vi "Main.vi"(11 "Module Admin":refnum<class "Delacor_lib_QMH_Module Admin.lvclass">) -> ()   [LabVIEW 2024, in "UI.lvlib"]
doc: "This template is based off of the Queued Message Handler design pattern and the Queued Message Handler project template that ships with LabVIEW.\n\nThe main difference is that the queue is private to this module and communication between modules is performed via Broadcast and Request events.\n\nRequest events are wrapped in public API methods and are handled in the Event Handling Loop (EHL) of this VI. Any module can register for Broadcast events sent by this module. The EHL generates messages based on user interface actions.\n\nThe Message Handling Loop (MHL) processes messages generated by the EHL, or by other messages. The messages are string values, so new messages can be added easily to the Message Cases case structure in the MHL. Each message cluster can also provide an optional value for Message Data, which is a variant that can be converted to whatever message-specific data is required.\n_____\nBased on DQMH Dev Tools: Project Template 7.1.0.1503."
uses:
  UI.lvlib
  <vilib>/Delacor/Delacor QMH/Libraries/Module Admin_class/Delacor_lib_QMH_Module Admin.lvclass
  Module Data--cluster.ctl
  Stop Argument--cluster.ctl
  <vilib>/Delacor/Delacor QMH/Libraries/Message Queue_class/Delacor_lib_QMH_Message Queue.lvclass/Delacor_lib_QMH_Message Queue.ctl
  <vilib>/Delacor/Delacor QMH/Libraries/Module Admin_class/Delacor_lib_QMH_Module Admin.lvclass/Delacor_lib_QMH_Module Admin.ctl
  <vilib>/Delacor/Delacor QMH/Libraries/Message Queue_class/Delacor_lib_QMH_Enqueue Message (Single).vi
  <vilib>/Delacor/Delacor QMH/Libraries/Module Admin_class/Delacor_lib_QMH_Get External Launch.vi
  <vilib>/Delacor/Delacor QMH/Libraries/Message Queue_class/Delacor_lib_QMH_Message Queue.lvclass
  <vilib>/PantherLAB/Message Module/Libraries/Message/PantherLAB_lib_Message.lvlib
  MoneyControl/MoneyControl.lvlib
  ProductControl/ProductControl.lvlib
panel:
  in  "Inventario Listbox":i32(listbox)
  out "Status":string
  in  "Comprar":bool
  out "error out":errorcluster
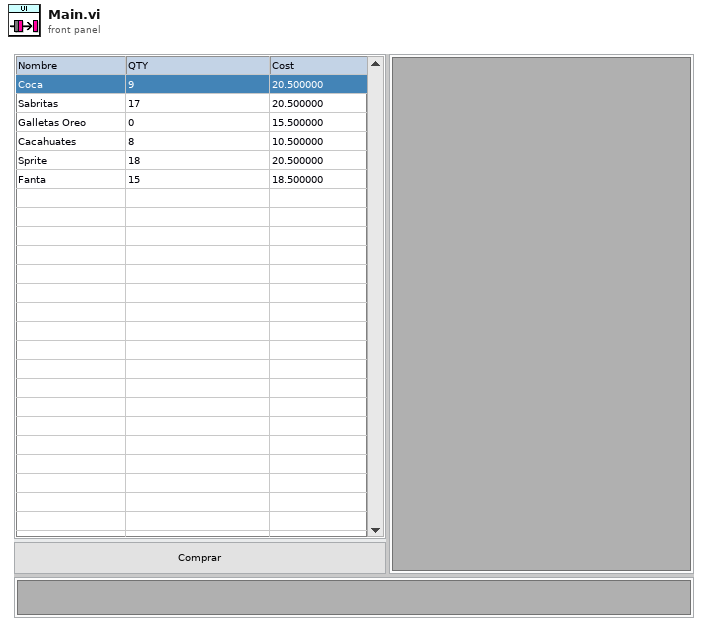
[diagram p1: front panel]
types:
  T1 = typedef "UI.lvlib/Request Events--cluster.ctl" = cluster{"Stop Module":refnum<user-event>, "Show Panel":refnum<user-event>, "Hide Panel":refnum<user-event>, "Get Module Execution Status":refnum<user-event>, "Show Diagram":refnum<user-event>, "Private.Lanza otros modulos":refnum<user-event>}
  T2 = typedef "PantherLAB_lib_Message.lvlib/Broadcast Events--cluster.ctl" = cluster{"Module Did Init":refnum<user-event>, "Status Updated":refnum<user-event>, "Error Reported":refnum<user-event>, "Module Did Stop":refnum<user-event>, "Update Module Execution Status":refnum<user-event>}
  T3 = typedef "MoneyControl.lvlib/Broadcast Events--cluster.ctl" = cluster{"Module Did Init":refnum<user-event>, "Status Updated":refnum<user-event>, "Error Reported":refnum<user-event>, "Module Did Stop":refnum<user-event>, "Update Module Execution Status":refnum<user-event>, "Credito Actualizado":refnum<user-event>, "Cambio Actualizado":refnum<user-event>}
  T4 = typedef "ProductControl.lvlib/Broadcast Events--cluster.ctl" = cluster{"Module Did Init":refnum<user-event>, "Status Updated":refnum<user-event>, "Error Reported":refnum<user-event>, "Module Did Stop":refnum<user-event>, "Update Module Execution Status":refnum<user-event>, "Inventario Actualizado":refnum<user-event>}
  T5 = typedef "UI.lvlib/Module Data--cluster.ctl" = cluster{"Status":string, "Message Module ID":i32}
  T6 = enum32{"invalid lock state", "Not Locked", "Locked (No Password)", "Password-protected"}
  T7 = typedef "UI.lvlib/Stop Argument--cluster.ctl" = cluster{"Origin":string, "Exit via Stop Module Req?":bool, "Wait for Module to stop?":bool}
  T8 = enum32{"Invalid", "Standard", "Closed", "Hidden", "Minimized", "Maximized"}
  T9 = typedef "ProductControl.lvlib/Products--array.ctl" = cluster{"Nombre":string, "QTY":u32, "Value":dbl}[]
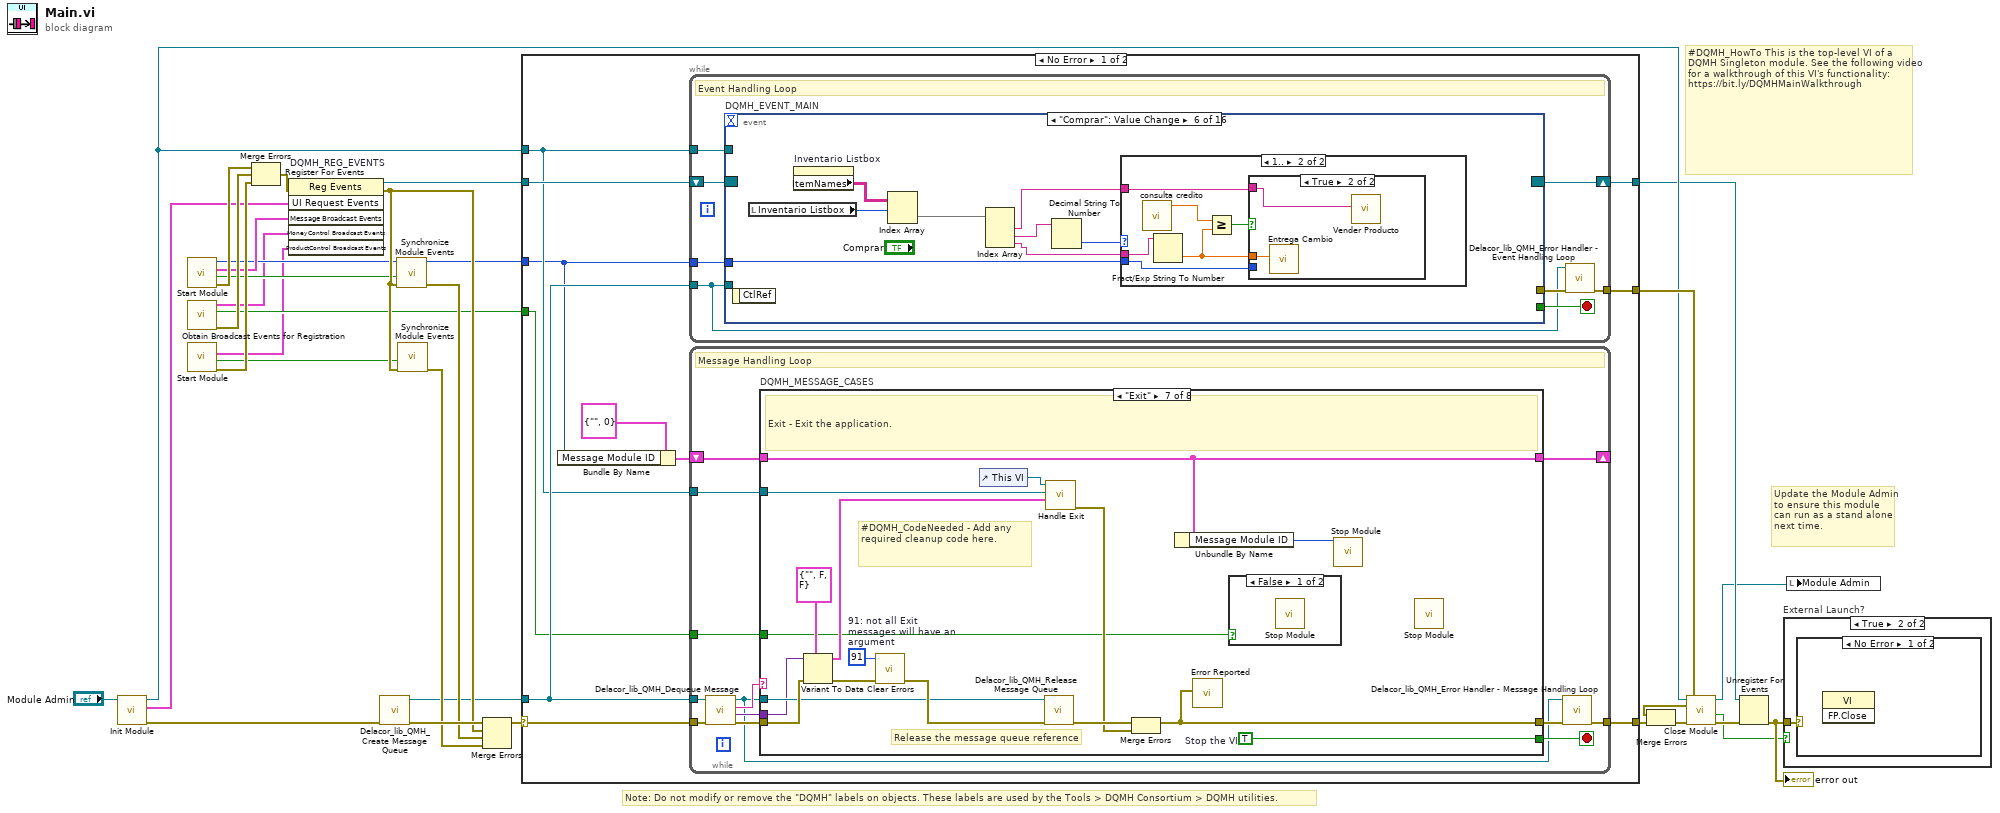
[diagram p0: block diagram]
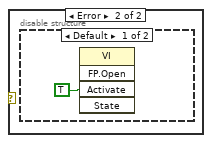
[diagram p3: hidden frame]
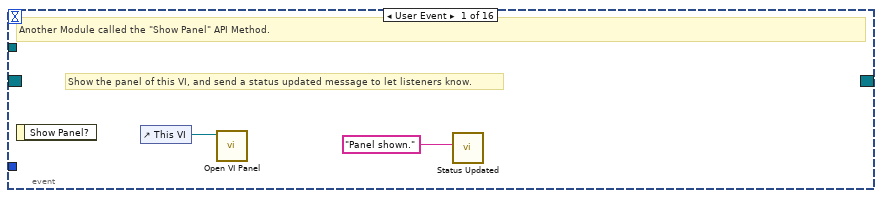
[diagram p5: hidden frame]
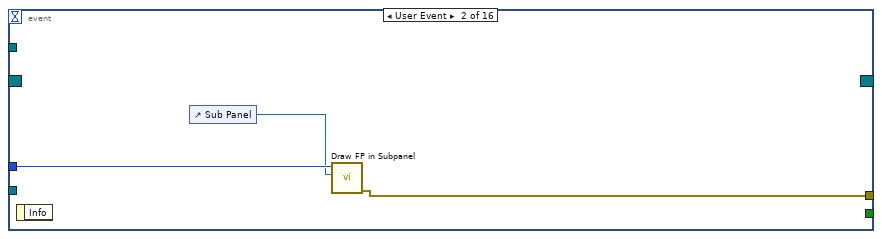
[diagram p6: hidden frame]
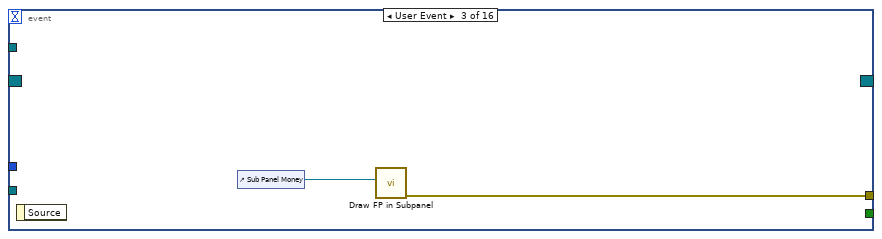
[diagram p7: hidden frame]
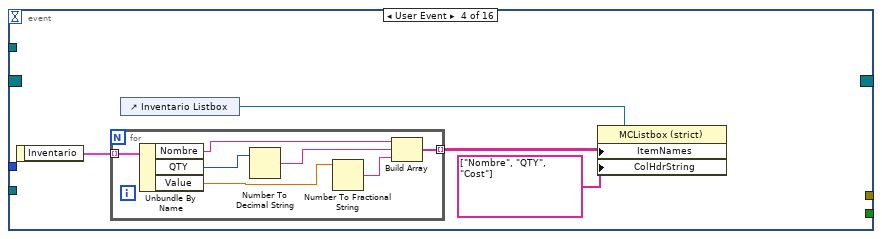
[diagram p8: hidden frame]
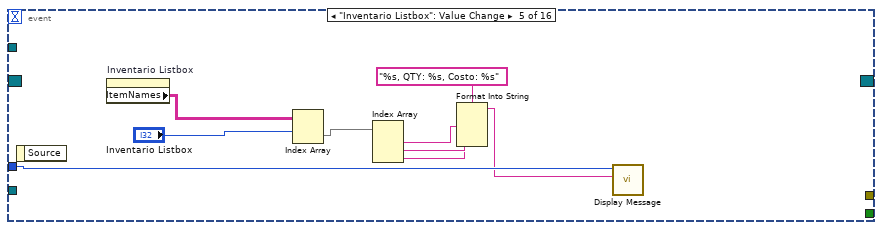
[diagram p9: hidden frame]
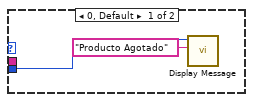
[diagram p10: hidden frame]
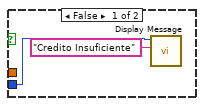
[diagram p11: hidden frame]
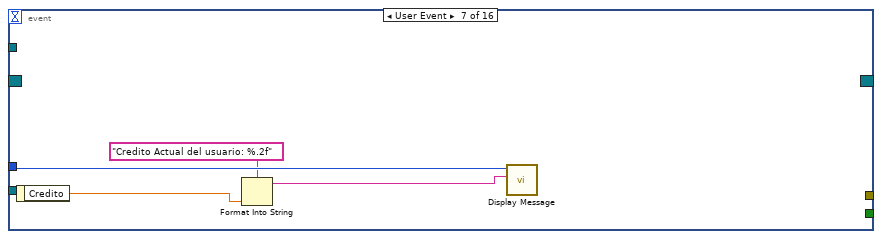
[diagram p12: hidden frame]
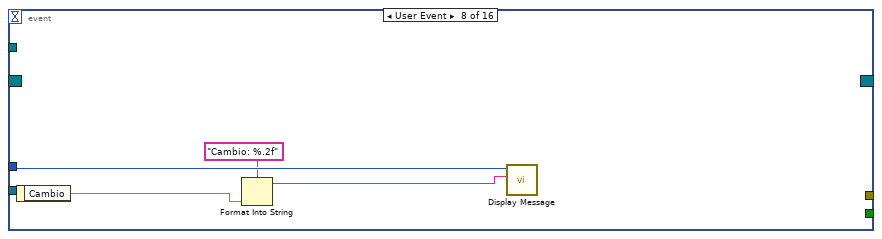
[diagram p13: hidden frame]
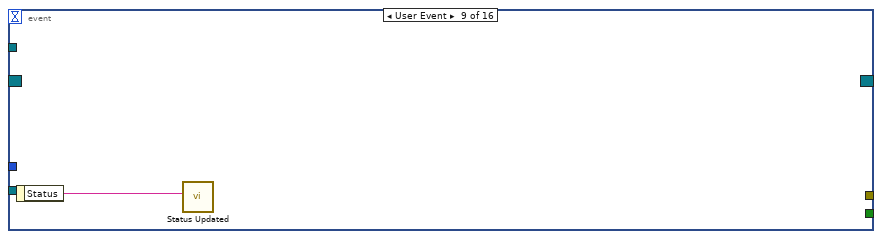
[diagram p14: hidden frame]
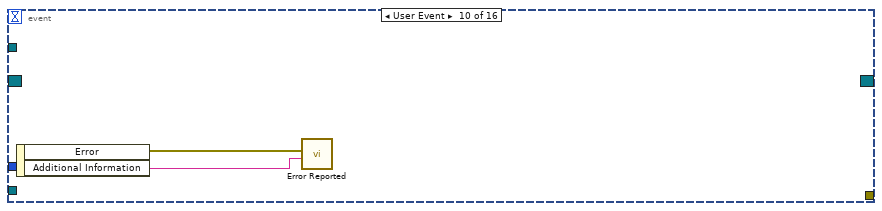
[diagram p15: hidden frame]
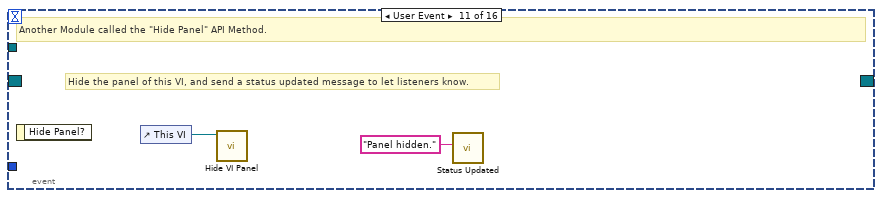
[diagram p16: hidden frame]
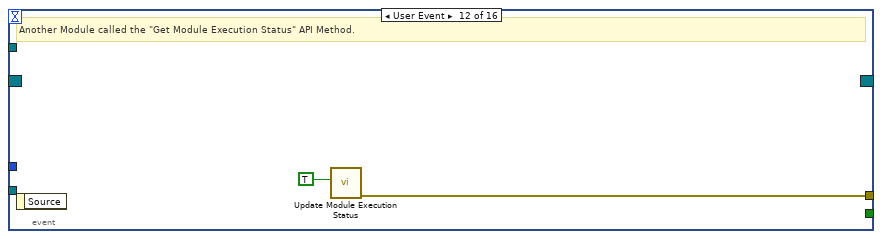
[diagram p17: hidden frame]
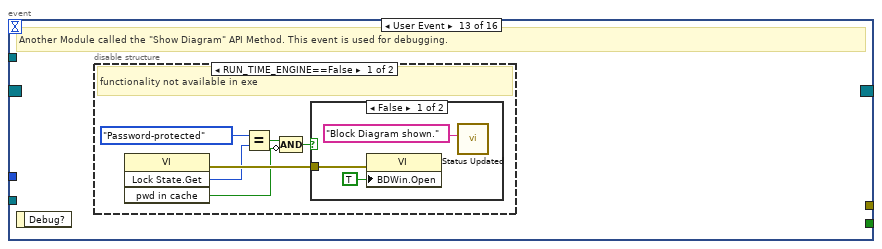
[diagram p18: hidden frame]
diagram:
  # "#DQMH_HowTo This is the top-level VI of a DQMH Singleton module. See the following video for a walkthrough of this VI's functionality: https://bit.ly/DQMHMainWalkthrough"
  # "Note: Do not modify or remove the \"DQMH\" labels on objects. These labels are used by the Tools > DQMH Consortium > DQMH utilities."
  # "Update the Module Admin to ensure this module can run as a stand alone next time."
  n1 = call "Init Module.vi"("Singleton Module Admin in"="Module Admin") -> ("error out"=w30:errorcluster, "UI Request Events"=w13:T1, "Singleton Module Admin out"=w16:refnum<class "Delacor_lib_QMH_Module Admin.lvclass">)  [unwired: 8 in]
  n2 = call <vilib>:"Start Module.vi"() -> ("error out"=w23:errorcluster, "Wait for Event Sync?"=w7:bool, "Message Broadcast Events"=w8:T2, "Module ID"=w6:i32)  [unwired: 7 in, 1 out]
  n3 = call "Obtain Broadcast Events for Registration.vi"() -> ("error out"=w20:errorcluster, "Already running?"=w3:bool, "MoneyControl Broadcast Events"=w4:T3)  [unwired: 9 in]
  n4 = call <vilib>:"Start Module.vi"() -> ("error out"=w19:errorcluster, "Wait for Event Sync?"=w1:bool, "ProductControl Broadcast Events"=w2:T4)  [unwired: 7 in, 2 out]
  n5 = Merge Errors(w23, w20, w19) -> (w22:errorcluster)
  n6 = register-events "DQMH_REG_EVENTS"(error in=w22, w13, w8, w4, w2) -> (reference out=w14:refnum<event-registration>, error out=w18:errorcluster)  [unwired: 1 in]
  n7 = call <vilib>:"Delacor_lib_QMH_Create Message Queue.vi"("error in"=w30) -> ("error out"=w25:errorcluster, "Message Queue"=w12:refnum<class "Delacor_lib_QMH_Message Queue.lvclass">)  [unwired: 9 in]
  n8 = call <vilib>:"Synchronize Module Events.vi"("error in"=w18, "Wait for Event Sync?"=w7, "Module ID in"=w6) -> ("error out"=w21:errorcluster, "Module ID out"=w5:i32)  [unwired: 7 in]
  n9 = call <vilib>:"Synchronize Module Events.vi"("error in"=w18, "Wait for Event Sync?"=w1) -> ("error out"=w17:errorcluster)  [unwired: 9 in]
  n10 = Merge Errors(w25, w18, w21, w17) -> (w24:errorcluster)
  n11 = case shown="No Error" w24 {
    selector: w24 -> [w40 w261]
    tunnel: [w42 w260] -> w31
    tunnel: [w39 w259] -> w15
    tunnel: w14 -> [w37 w259]
    tunnel: w12 -> [w36 w255]
    tunnel: [w41 _] -> w28
    tunnel: w16 -> [w35 w256]
    tunnel: w5 -> [w33 w254]
    tunnel: w3 -> [w32 w253]
    frame No Error {
      n12 = Bundle By Name(cluster=T5 {"Status"="", "Message Module ID"=0} ("Data Cluster"), "Message Module ID"=w33) -> (w34:T5)
      n13 = while {
        tunnel: w36 -> [w44]
        shift-right: [w47] -> w39
        shift-left: w37 -> [w48]
        tunnel: [w49] -> w41
        tunnel: w35 -> [w45]
        tunnel: w33 -> [w43]
        stop <- w46 stop-if-true
        # "Event Handling Loop"
        n14 = event "DQMH_EVENT_MAIN" shown="[5] \"Comprar\": Value Change" {
          selector: w48 -> [_ _ _ _ _ _ _ _ _ _ _ _ _ _ _ w150]
          dyn-events: [_ _ _ _ _ _ _ _ _ _ _ _ _ _ _ w149] -> w47
          timeout: _ -> [_ _ _ _ _ _ _ _ _ _ _ _ _ _ _ _]
          tunnel: [_ _ _ _ _ _ _ _ _ _ _ _ _ TRUE ("Discard?") _ _] -> w46
          tunnel: w44 -> [_ _ _ _ _ _ _ _ _ _ _ _ _ w129 w136 _]
          tunnel: [_ w55 w57 _ _ _ _ _ _ _ _ w112 _ w132 w138 w151] -> w50
          tunnel: w45 -> [_ _ _ _ _ _ _ _ _ _ _ _ _ _ w135 _]
          tunnel: w43 -> [_ w54 _ _ w71 w81 w101 w105 _ _ _ _ _ _ _ _]
          event User Event {
            # "Show the panel of this VI, and send a status updated message to let listeners know."
            # "Another Module called the \"Show Panel\" API Method."
            n15 = event-data() -> ()  [unwired: 1 in, 1 out]
            n16 = control-ref of="This VI"() -> (w52:refnum<vi>)
            n17 = call "Open VI Panel.vi"("VI"=w52) -> ()  [unwired: 10 in, 1 out]
            n18 = call "Status Updated.vi"("Status"="Panel shown." ("format string")) -> ()  [unwired: 10 in, 1 out]
          }
          event User Event {
            n19 = event-data() -> ()  [unwired: 1 in, 1 out]
            n20 = control-ref of="Sub Panel"() -> (w53:refnum<vi>)
            n21 = call <vilib>:"Draw FP in Subpanel.vi"("Sub Panel"=w53, "Module ID"=w54) -> ("error out"=w55:errorcluster)  [unwired: 9 in]
          }
          event User Event {
            n22 = event-data() -> ()  [unwired: 1 in, 1 out]
            n23 = control-ref of="Sub Panel Money"() -> (w56:refnum<vi>)
            n24 = call <vilib>:"Draw FP in Subpanel.vi"("Sub Panel"=w56) -> ("error out"=w57:errorcluster)  [unwired: 10 in]
          }
          event User Event {
            n25 = event-data() -> ("Inventario"=w60:T9)  [unwired: 1 in]
            n26 = for {
              tunnel: w60 -> [w68] mode=indexing
              tunnel: [w62] -> w59 mode=indexing
              n27 = Unbundle By Name(w68) -> ("Nombre"=w65:string, "QTY"=w67:u32, "Value"=w66:dbl)
              n28 = Number To Decimal String(number=w67) -> (decimal integer string=w64:string)  [unwired: 1 in]
              n29 = Number To Fractional String(number=w66) -> (F-format string=w63:string)  [unwired: 3 in]
              n30 = Build Array(w65, w64, w63) -> (w62:string[])
            }
            n31 = control-ref of="Inventario Listbox"() -> (w61:refnum<vi>)
            n32 = property class="MCListbox (strict)"(reference=w61, "ItemNames"=w59, "ColHdrString"=string[] ["Nombre", "QTY", "Cost"] ("Column Header Strings[]")) -> ()  [unwired: 1 in, 2 out]
          }
          event "Inventario Listbox": Value Change {
            n33 = event-data() -> ()  [unwired: 1 in, 1 out]
            n34 = property on="Inventario Listbox" class="MCListbox (strict)"() -> ("ItemNames"=w77:string[][])  [unwired: 2 in, 2 out]
            n35 = Index Array(array=w77, index (row)="Inventario Listbox") -> (element=w75:string[])  [unwired: 1 in]
            n36 = Index Array(array=w75) -> (element #1=w74:string, element #2=w73:string, element #3=w72:string)  [unwired: 3 in]
            n37 = Format Into String(format string="%s, QTY: %s, Costo: %s", w74, w73, w72) -> (resulting string=w70:string)  [unwired: 2 in, 1 out]
            n38 = call <vilib>:"Display Message.vi"("Message"=w70, "Module ID"=w71) -> ()  [unwired: 9 in, 1 out]
          }
          event "Comprar": Value Change {
            n39 = event-data() -> ()  [unwired: 1 in, 1 out]
            n40 = local read "Inventario Listbox"() -> (w85:i32)
            n41 = property on="Inventario Listbox" class="MCListbox (strict)"() -> ("ItemNames"=w84:string[][])  [unwired: 2 in, 2 out]
            n42 = Index Array(array=w84, index (row)=w85) -> (element=w83:string[])  [unwired: 1 in]
            n43 = Index Array(array=w83) -> (element #1=w78:string, element #2=w79:string, element #3=w80:string)  [unwired: 3 in]
            n44 = Decimal String To Number(string=w79) -> (number=w82:i32)  [unwired: 2 in, 1 out]
            n45 = case shown="1.." w82 {
              tunnel: w81 -> [w87 w89]
              tunnel: w80 -> [_ w93]
              tunnel: w78 -> [_ w88]
              frame 0, Default {
                n46 = call <vilib>:"Display Message.vi"("Message"="Producto Agotado", "Module ID"=w87) -> ()  [unwired: 9 in, 1 out]
              }
              frame 1.. {
                n47 = call "consulta credito.vi"() -> ("Credito Actual"=w90:dbl)  [unwired: 9 in, 2 out]
                n48 = Fract/Exp String To Number(string=w93) -> (number=w91:dbl)  [unwired: 3 in, 1 out]
                n49 = Greater Or Equal?(x=w90, y=w91) -> (x >= y?=w92:bool)
                n50 = case shown="True" w92 {
                  tunnel: w91 -> [_ w97]
                  tunnel: w89 -> [w94 _]
                  tunnel: w88 -> [_ w96]
                  frame False {
                    n51 = call <vilib>:"Display Message.vi"("Message"="Credito Insuficiente", "Module ID"=w94) -> ()  [unwired: 9 in, 1 out]
                  }
                  frame True {
                    n52 = call "Entrega Cambio.vi"("Valor Producto"=w97) -> ()  [unwired: 10 in, 1 out]
                    n53 = call "Vender Producto.vi"("Nombre Producto"=w96) -> ()  [unwired: 10 in, 1 out]
                  }
                }
              }
            }
          }
          event User Event {
            n54 = event-data() -> ("Credito"=w100:dbl)  [unwired: 1 in]
            n55 = Format Into String(format string="Credito Actual del usuario: %.2f", w100) -> (resulting string=w99:string)  [unwired: 2 in, 1 out]
            n56 = call <vilib>:"Display Message.vi"("Message"=w99, "Module ID"=w101) -> ()  [unwired: 9 in, 1 out]
          }
          event User Event {
            n57 = event-data() -> ("Cambio"=w104:dbl)  [unwired: 1 in]
            n58 = Format Into String(format string="Cambio: %.2f", w104) -> (resulting string=w103:string)  [unwired: 2 in, 1 out]
            n59 = call <vilib>:"Display Message.vi"("Message"=w103, "Module ID"=w105) -> ()  [unwired: 9 in, 1 out]
          }
          event User Event {
            n60 = event-data() -> ("Status"=w106:string)  [unwired: 1 in]
            n61 = call "Status Updated.vi"("Status"=w106) -> ()  [unwired: 10 in, 1 out]
          }
          event User Event {
            n62 = event-data() -> ("Error"=w108:errorcluster, "Additional Information"=w107:string)  [unwired: 1 in]
            n63 = call "Error Reported.vi"("Additional Information"=w107, "Error"=w108) -> ()  [unwired: 9 in, 1 out]
          }
          event User Event {
            # "Hide the panel of this VI, and send a status updated message to let listeners know."
            # "Another Module called the \"Hide Panel\" API Method."
            n64 = event-data() -> ()  [unwired: 1 in, 1 out]
            n65 = control-ref of="This VI"() -> (w110:refnum<vi>)
            n66 = call "Hide VI Panel.vi"("VI"=w110) -> ()  [unwired: 10 in, 1 out]
            n67 = call "Status Updated.vi"("Status"="Panel hidden." ("format string")) -> ()  [unwired: 10 in, 1 out]
          }
          event User Event {
            # "Another Module called the \"Get Module Execution Status\" API Method."
            n68 = event-data() -> ()  [unwired: 1 in, 1 out]
            n69 = call "Update Module Execution Status.vi"("Running?"=TRUE) -> ("error out"=w112:errorcluster)  [unwired: 10 in]
          }
          event User Event {
            # "Another Module called the \"Show Diagram\" API Method. This event is used for debugging."
            n70 = event-data() -> ()  [unwired: 1 in, 1 out]
            n71 = disable-structure shown="RUN_TIME_ENGINE==False" {
              frame condition #0 (active) {
                # "functionality not available in exe"
                n72 = invoke on="Invoke Node" class="VI" method="Lock State.Get"() -> (error out=w118:errorcluster, "Get Lock State"=w117:T6, "pwd in cache"=w114:bool)  [unwired: 4 in, 1 out]
                n73 = Equal?(x=T6."Password-protected", y=w117) -> (x = y?=w115:bool)
                n74 = Compound Arithmetic op=AND(w115, invert w114) -> (w113:bool)
                n75 = case shown="False" w113 {
                  tunnel: w118 -> [w121 _]
                  frame False {
                    n76 = property on="Property Node" class="VI"(error in=w121, "BDWin.Open"=TRUE ("Block Diagram Window:Open")) -> ()  [unwired: 1 in, 2 out]
                    n77 = call "Status Updated.vi"("Status"="Block Diagram shown." ("format string")) -> ()  [unwired: 10 in, 1 out]
                  }
                  frame True {
                    # "Password-protected VI, and the password is not in the cache. Do not show the diagram."
                  }
                }
              }
              frame condition #1 {
              }
            }
          }
          event User Event {
            # "The Stop Module Event can get fired from the Exit message in the MHL. The queue gets destroyed in that case. If the queue no longer exists, the Enqueue Exit as a priority message will return error 1. It is safe to ignore, because the module is already exiting."
            # "Another Module called the \"Stop Module\" API Method  or the Message Handling Loop below."
            n78 = event-data() -> ("Origin"=w128:string, "Exit via Stop Module Req?"=w124:bool, "Wait for Module to stop?"=w123:bool)  [unwired: 1 in]
            n79 = local write "Status"(w128) -> ()
            n80 = Bundle By Name(cluster=T7 {"Origin"="", "Exit via Stop Module Req?"=FALSE, "Wait for Module to stop?"=FALSE} ("Stop Argument"), "Exit via Stop Module Req?"=w124, "Wait for Module to stop?"=w123) -> (w122:T7)
            n81 = call-poly <vilib>:"Delacor_lib_QMH_Enqueue Message (poly).vi"("Priority Message? (F)"=TRUE, "Message Data"=w122, "Message"="Exit", "Message Queue in"=w129) -> ("error out"=w133:errorcluster)  [unwired: 6 in, 1 out]
            n82 = call <vilib>:"Clear Errors.vi"("error in (no error)"=w133, "specific error code to clear (0: all)"=1) -> ("error out"=w132:errorcluster)  [unwired: 4 in, 1 out]
          }
          event Panel Close? {
            w137 = TRUE  # Discard the event, the MHL is responsible for closing and stopping this VI.
            # "Hide the panel or send the 'Exit' message if the user clicks the 'X' on the module main VI panel."
            n83 = event-data() -> ()  [unwired: 1 in, 1 out]
            n84 = property on="Property Node" class="Module Admin"(reference=w135) -> ("Accessors:External Launch"=w134:bool)  [unwired: 1 in, 2 out]
            n85 = case shown="True" w134 {
              tunnel: w136 -> [_ w144]
              tunnel: [_ w145] -> w138
              frame True {
                # "If externally launched, clicking the 'X' hides the panel, but doesn't close it."
                n86 = control-ref of="This VI"() -> (w140:refnum<vi>)
                n87 = call "Hide VI Panel.vi"("VI"=w140) -> ("error out"=w141:errorcluster)  [unwired: 10 in]
                n88 = call "Status Updated.vi"("error in"=w141, "Status"="Panel hidden." ("format string")) -> ()  [unwired: 9 in, 1 out]
              }
              frame False {
                # "If run as a stand-alone VI, clicking the panel 'X' stops the VI."
                n89 = call-poly <vilib>:"Delacor_lib_QMH_Enqueue Message (poly).vi"("Priority Message? (F)"=TRUE, "Message"="Exit", "Message Queue in"=w144) -> ("error out"=w145:errorcluster)  [unwired: 7 in, 1 out]
              }
            }
            n90 = event-data ("Event Filter Node")("Discard?"=w137) -> ()  [unwired: 1 in, 1 out]
          }
          event User Event {
            # "This module called the \"Private.Lanza otros modulos\" private request."
            n91 = event-data() -> ()  [unwired: 1 in, 1 out]
            n92 = call <vilib>:"Start Module.vi"() -> ("error out"=w153:errorcluster, "Wait for Event Sync?"=w148:bool, "MoneyControl Broadcast Events"=w147:T3, "Module Was Already Running?"=w146:bool)  [unwired: 7 in, 1 out]
            n93 = register-events(reference=w150, error in=w153, w147) -> (reference out=w149:refnum<event-registration>, error out=w154:errorcluster)  [unwired: 3 in]
            n94 = call <vilib>:"Synchronize Module Events.vi"("error in"=w154, "Wait for Event Sync?"=w148) -> ("error out"=w152:errorcluster)  [unwired: 9 in]
            n95 = case shown="False" w146 {
              tunnel: w152 -> [w155 w158]
              tunnel: [w155 w157] -> w151
              frame False {
              }
              frame True {
                n96 = control-ref of="Sub Panel Money"() -> (w156:refnum<vi>)
                n97 = call <vilib>:"Draw FP in Subpanel.vi"("error in"=w158, "Sub Panel"=w156) -> ("error out"=w157:errorcluster)  [unwired: 9 in]
              }
            }
          }
        }
        n98 = call-dynamic "Delacor_lib_QMH_Error Handler - Event Handling Loop.vi"("error in"=w50, "Message Queue in"=w44) -> ("dup error in"=w49:errorcluster)  [unwired: 8 in, 1 out]
      }
      n99 = while {
        tunnel: w36 -> [w160]
        shift-right: [w166] -> _
        shift-left: w34 -> [w167]
        tunnel: w40 -> [w171]
        tunnel: [w169] -> w42
        tunnel: w35 -> [w162]
        tunnel: w32 -> [w159]
        stop <- w165 stop-if-true
        # "Message Handling Loop"
        n100 = call-dynamic "Delacor_lib_QMH_Dequeue Message.vi"("error in"=w171, "Message Queue in"=w160) -> ("error out"=w170:errorcluster, "Message Data"=w163:variant, "Message"=w164:string, "Message Queue out"=w161:refnum<class "Delacor_lib_QMH_Message Queue.lvclass">)  [unwired: 6 in]
        n101 = case "DQMH_MESSAGE_CASES" shown="\"Exit\"" w164 {
          selector: w164 -> [_ _ _ _ _ _ _ w247]
          tunnel: w161 -> [_ _ _ _ _ w210 w235 _]
          tunnel: w170 -> [w189 w193 w196 w198 w207 w218 w241 w250]
          tunnel: [w186 w193 w195 w198 w206 w214 w236 w251] -> w168
          tunnel: w167 -> [w177 w192 w194 w197 w204 w212 w227 w248]
          tunnel: [w176 w192 w194 w197 w204 w212 w227 w248] -> w166
          tunnel: [_ _ _ _ _ _ w234 _] -> w165
          tunnel: w163 -> [_ _ _ _ _ w211 w233 _]
          tunnel: w162 -> [w178 _ _ _ _ w209 w228 _]
          tunnel: w159 -> [_ _ _ _ _ _ w225 _]
          frame "Initialize" {
            w172 = "Initial Message" ("Initial Message")
            # "Initialize - Any operation that needs to be done before the module can receive messages. Synchronize Caller Events.vi will inform Start Module.vi that the module has launched and is ready to receive messages. Module Did Init.vi will broadcast that the module initialized."
            n102 = call "Synchronize Caller Events.vi"("error in"=w189, "Singleton Module Admin in"=w178) -> ("error out"=w188:errorcluster, "Singleton Module Admin out"=w173:refnum<class "Delacor_lib_QMH_Module Admin.lvclass">)  [unwired: 8 in]
            n103 = property on="Property Node" class="Module Admin"(reference=w173) -> ("Accessors:External Launch"=w182:bool)  [unwired: 1 in, 2 out]
            n104 = Select(t=T8."Hidden" ("State"), s=w182, f=T8."Standard" ("State")) -> (s? t:f=w179:T8)
            n105 = call "Module Name--constant.vi"() -> ("Module Name"=w185:string)  [unwired: 11 in]
            n106 = property on="Property Node" class="VI"("Front Panel.Title"=w185) -> (reference out=w184:refnum<vi>, error out=w191:errorcluster)  [unwired: 2 in]
            n107 = invoke on="Invoke Node" class="VI" method="FP.Open"(reference=w184, error in=w191, "State"=w179) -> (reference out=w183:refnum<vi>, error out=w190:errorcluster)  [unwired: 2 in, 3 out]
            n108 = Bundle By Name(cluster=w177, "Status"=w172) -> (w176:T5)
            n109 = invoke on="Invoke Node" class="VI" method="FP.Center"(reference=w183, error in=w190) -> ()  [unwired: 1 in, 3 out]
            n110 = call "Module Name--constant.vi"() -> ("Module Name"=w174:string)  [unwired: 11 in]
            n111 = call "Module Did Init.vi"("error in"=w188, "Initialized?"=TRUE, "Origin"=w174) -> ("error out"=w187:errorcluster)  [unwired: 8 in]
            n112 = call "Lanza otros modulos.vi"("error in"=w187) -> ("error out"=w186:errorcluster)  [unwired: 10 in]
            "Status" <- w172
          }
          frame "---Module Specific---" {
            # "Separator -- The following cases handle messages specific to this Module."
          }
          frame "---Copy This Frame---" {
            # "Duplicate this frame when creating new messages.  Change this comment in the duplicated frame to describe this message."
            n113 = Merge Errors(w196) -> (w195:errorcluster)
          }
          frame "---Exit and Error Handling---" {
            # "Separator - The following cases handle errors and exit messages."
          }
          frame "Simulate MHL Error" {
            # "#DQMH_HowTo The 'Simulate MHL Error' button  illustrates how the MHL handles errors. This event is instructional in nature and can be removed."
            # "Simulate an error occurring at the MHL"
            n114 = call "Module Name--constant.vi"() -> ("Module Name"=w200:string)  [unwired: 11 in]
            n115 = Format Into String(format string="Simulated error originating at Message Handling Loop in %s", w200) -> (resulting string=w201:string)  [unwired: 2 in, 1 out]
            n116 = call <vilib>:"Error Cluster From Error Code.vi"("show call chain? (False)"=TRUE, "error message (\"\")"=w201, "error code (0)"=5001) -> ("error out"=w205:errorcluster)  [unwired: 6 in]
            n117 = Merge Errors(w207, w205) -> (w206:errorcluster)
          }
          frame "Error" {
            # "#DQMH_CodeRecommended - If the module is running in standalone mode (External Launch = FALSE), this code will pop up an error dialog and call the 'Exit' message if an error occurs. Add more fine-grained error management here."
            # "Error - Check the error message data and respond accordingly. This message is sent by the \"Error Handler\" VIs at the end of each loop in this application."
            n118 = property on="Property Node" class="Module Admin"(reference=w209) -> ("Accessors:External Launch"=w208:bool)  [unwired: 1 in, 2 out]
            n119 = Variant To Data(error in=w218, type=errorcluster {"status"=FALSE, "code"=0, "source"=""} ("error constant"), Variant=w211) -> (data=w213:errorcluster, error out=w216:errorcluster)
            n120 = local write "error out"(w213) -> ()
            n121 = call "Error Reported.vi"("Error"=w213) -> ()  [unwired: 10 in, 1 out]
            n122 = case shown="False" w208 {
              tunnel: [w223 _] -> w215
              tunnel: w210 -> [w221 _]
              tunnel: w213 -> [w222 _]
              frame False {
                n123 = disable-structure shown="Default" {
                  disable-tunnel: w222 -> [w224 _]
                  frame condition #0 (active) {
                    # "If the module is running standalone, then pop up an error dialog and call the \"Exit\" message."
                    n124 = call <vilib>:"Simple Error Handler.vi"("error in (no error)"=w224) -> ()  [unwired: 4 in, 5 out]
                  }
                  frame condition #1 {
                    # "To prevent the Simple Error Handler VI from being loaded (e.g. when deploying to a Real-Time target), add the Conditional Disable Symbol \"DQMH_Disable_SEH\" to your project and set it to TRUE."
                  }
                }
                n125 = call-poly <vilib>:"Delacor_lib_QMH_Enqueue Message (poly).vi"("Priority Message? (F)"=TRUE, "Message"="Exit", "Message Queue in"=w221) -> ("error out"=w223:errorcluster)  [unwired: 7 in, 1 out]
              }
              frame True {
                # "If the module was launched externally, calling the Error Reported broadcast VI is the only action performed by the \"Error\" message. The module's caller can then process the error appropriately."
              }
            }
            n126 = Merge Errors(w216, w215) -> (w214:errorcluster)
          }
          frame "Exit" {
            w232 = 91  # 91: not all Exit messages will have an argument
            w234 = TRUE  # Stop the VI
            # "Release the message queue reference"
            # "#DQMH_CodeNeeded - Add any required cleanup code here."
            # "Exit - Exit the application."
            n127 = Variant To Data(error in=w241, type=T7 {"Origin"="", "Exit via Stop Module Req?"=FALSE, "Wait for Module to stop?"=FALSE} ("Stop Argument"), Variant=w233) -> (data=w230:T7, error out=w238:errorcluster)
            n128 = call <vilib>:"Clear Errors.vi"("error in (no error)"=w238, "specific error code to clear (0: all)"=w232) -> ("error out"=w240:errorcluster)  [unwired: 4 in, 1 out]
            n129 = control-ref of="This VI"() -> (w229:refnum<vi>)
            n130 = call-dynamic "Delacor_lib_QMH_Release Message Queue.vi"("error in"=w240, "Message Queue"=w235) -> ("error out"=w239:errorcluster)  [unwired: 9 in]
            n131 = call "Handle Exit.vi"("Stop Argument"=w230, "Admin in"=w228, "VI reference"=w229) -> ("error out"=w237:errorcluster)  [unwired: 7 in, 1 out]
            n132 = Merge Errors(w239, w237) -> (w236:errorcluster)
            n133 = Unbundle By Name(w227) -> ("Message Module ID"=w226:i32)
            n134 = call "Error Reported.vi"("Error"=w236) -> ()  [unwired: 10 in, 1 out]
            n135 = case shown="False" w225 {
              frame False {
                n136 = call <vilib>:"Stop Module.vi"() -> ()  [unwired: 11 in, 1 out]
              }
              frame True {
              }
            }
            n137 = call <vilib>:"Stop Module.vi"("Module ID"=w226) -> ()  [unwired: 10 in, 1 out]
            n138 = call <vilib>:"Stop Module.vi"() -> ()  [unwired: 11 in, 1 out]
          }
          frame Default {
            # "'Default' case only runs if there is a message that isn't defined in any of the other cases.  Output a programming error."
            n139 = call "Module Name--constant.vi"() -> ("Module Name"=w246:string)  [unwired: 11 in]
            n140 = Format Into String(format string="The invalid message string \"%s\" was received in the Message Handling Loop for module \"%s\".", w247, w246) -> (resulting string=w242:string)  [unwired: 2 in, 1 out]
            n141 = call <vilib>:"Error Cluster From Error Code.vi"("show call chain? (False)"=TRUE, "error message (\"\")"=w242, "error code (0)"=1) -> ("error out"=w249:errorcluster)  [unwired: 6 in]
            n142 = Merge Errors(w250, w249) -> (w251:errorcluster)
          }
        }
        n143 = call-dynamic "Delacor_lib_QMH_Error Handler - Message Handling Loop.vi"("error in"=w168, "Message Queue in"=w161) -> ("dup error in"=w169:errorcluster)  [unwired: 8 in, 1 out]
      }
    }
    frame Error {
      # "Synchronize Caller Events.vi will inform Start Module.vi that the module has launched and will let the code calling Start Module.vi register for broadcasts and would permit the caller receive the broadcast that an error occurred at launch time."
      n144 = call-dynamic "Delacor_lib_QMH_Release Message Queue.vi"("error in"=w261, "Message Queue"=w255) -> ("error out"=w260:errorcluster)  [unwired: 9 in]
      n145 = call "Synchronize Caller Events.vi"("Singleton Module Admin in"=w256) -> ("error out"=w262:errorcluster)  [unwired: 9 in, 1 out]
      n146 = call "Module Name--constant.vi"() -> ("Module Name"=w258:string)  [unwired: 11 in]
      n147 = Format Into String(format string="An error occurred during initialization. %s is no longer running.", w258) -> (resulting string=w252:string)  [unwired: 2 in, 1 out]
      n148 = Merge Errors(w260, w262) -> (w263:errorcluster)
      n149 = case shown="False" w253 {
        tunnel: w252 -> [w264 _]
        frame False {
          n150 = call <vilib>:"Stop Module.vi"("Origin"=w264) -> ()  [unwired: 10 in, 1 out]
        }
        frame True {
        }
      }
      n151 = call "Error Reported.vi"("Additional Information"=w252, "Error"=w263) -> ()  [unwired: 9 in, 1 out]
      n152 = call <vilib>:"Stop Module.vi"("Origin"=w252) -> ()  [unwired: 10 in, 1 out]
      n153 = call <vilib>:"Stop Module.vi"("Origin"=w252, "Module ID"=w254) -> ()  [unwired: 9 in, 1 out]
    }
  }
  n154 = Merge Errors(w28, w31) -> (w27:errorcluster)
  n155 = call "Close Module.vi"("error in"=w27, "Module Admin in"=w16) -> ("error out"=w29:errorcluster, "External Launch"=w9:bool, "Module Admin out"=w10:refnum<class "Delacor_lib_QMH_Module Admin.lvclass">)  [unwired: 7 in]
  n156 = Unregister For Events(event registration refnum=w15, error in=w29) -> (error out=w26:errorcluster)
  "error out" <- w26
  n157 = case "External Launch?" shown="True" w9 {
    tunnel: w26 -> [_ w265]
    frame False {
    }
    frame True {
      n158 = case shown="No Error" w265 {
        frame No Error {
          n159 = invoke on="Invoke Node" class="VI" method="FP.Close"() -> ()  [unwired: 3 in, 3 out]
        }
        frame Error {
          n160 = disable-structure shown="Default" {
            frame condition #0 (active) {
              n161 = invoke class="VI" method="FP.Open"("Activate"=TRUE ("Activate?")) -> ()  [unwired: 4 in, 5 out]
            }
            frame condition #1 {
              # "Don't show panel on error if running inside a built EXE."
            }
          }
        }
      }
    }
  }
  n162 = local write "Module Admin"(w10) -> ()
